vi "Standard Engine.vi"(8 "error in":errorcluster, 11 "Engine Process Init Data":T1) -> (0 "error out":errorcluster)   [LabVIEW 2013, in "Standard Engine Runtime.lvclass"]
uses:
  Standard Engine Runtime.lvclass
  Engine Process Init Data.ctl
  Commands.ctl
  Engine Config Data.ctl
  Configuration/Standard Engine Configuration.lvclass
  <vilib>/NI/Tag Bus Module Framework/runtime/TBM module execution interface.lvclass
  <vilib>/NI/Tag Bus Module Framework/module configuration/TBM module configuration.lvclass
  <vilib>/NI/Module Execution Interface/Engine Runtime/Execution States.ctl
  <vilib>/Platform/TimedLoop/XDataNode/timing_clust.ctl
  <vilib>/Platform/TimedLoop/XDataNode/nitl_modes.ctl
  <vilib>/Platform/TimedLoop/XDataNode/wakeup.ctl
  <vilib>/NI/Module Timing Source/timing source/TBM timing source.lvclass/TBM timing source.ctl
  <vilib>/NI/Module Timing Source/timing source/TBM timing source.lvclass
  <vilib>/NI/Tag Bus/table/transfer table data.vi
  Module Execution Decimation.vi
  Error Handler.vi
  <vilib>/Utility/error.llb/Clear Errors.vi
  Delete Module Index.vi
  <vilib>/platform/TimedLoop/XDataNode/XDataNode.xnode
  <vilib>/NI/Module Execution Interface/Engine Runtime/Engine Runtime Interface.lvclass
  <vilib>/Platform/TimedLoop/XDataNode/XDNodeRunTimeDep.lvlib
panel:
  out "late?":bool
  out "iterations":i32
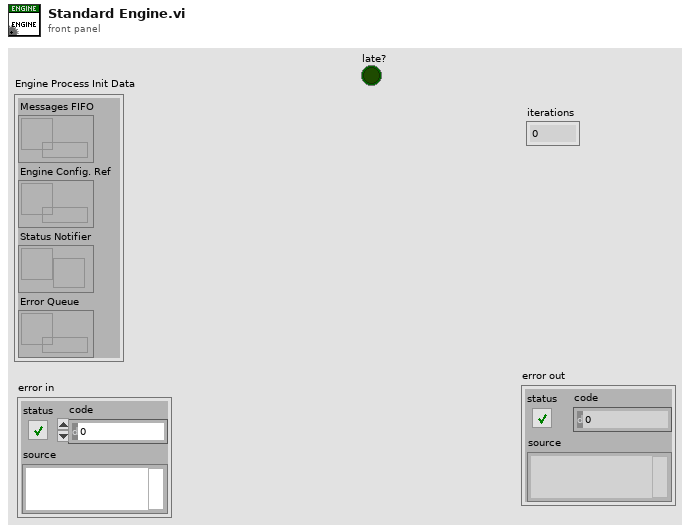
[diagram p1: front panel]
types:
  T1 = typedef "Standard Engine Runtime.lvclass/Engine Process Init Data.ctl" = cluster{"Messages FIFO":refnum<k33>, "Engine Config. Ref":refnum<data-value>, "Status Notifier":refnum<notifier>, "Error Queue":refnum<queue>}
  T2 = typedef "Engine Runtime Interface.lvclass/Execution States.ctl" = enum16{"Initializing", "Paused (Initialized)", "Running", "Set Safe Outputs", "Uninitializing", "Stopped (Uninitialized)", "Error (Uninitialized)", "Safe State (Uninitialized)", "Closed"}
  T3 = typedef "Standard Engine Runtime.lvclass/Commands.ctl" = enum16{"Initialize", "Start", "Pause", "Safe State", "Normal", "Stop", "Shutdown"}
  T4 = typedef "XDNodeRunTimeDep.lvlib/timing_clust.ctl" = cluster{"Expected End [f-1]":u64, "Actual End [f-1]":u64, "Finished Late? [f-1]":bool, "Expected End [i-1]":u64, "Actual End [i-1]":u64, "Finished Late? [i-1]":bool, "Expected Start [i]":u64, "Actual Start [i]":u64, "Expected Start [f]":u64, "Actual Start [f]":u64, "Source Name":string, "Structure Name":string, "Period":i64, "Deadline":i64, "Offset":i64, "Start":i64, "Priority":i32, "Timeout":i32, "Mode":T5, "Wakeup Reason":T6, "Error":errorcluster, "Source Type":string, "Secondary Source Type":string, "Global End Time":u64, "Global Start Time":u64, "Frame Duration":u64, "Iteration Duration":u64, "Assigned CPU":i32, "I/O Scan Engine Mode":u32}
  T5 = typedef "XDNodeRunTimeDep.lvlib/nitl_modes.ctl" = enum32{"No Change", "Process missed periods, maintain original phase", "Discard missed periods, maintain original phase", "Process missed periods, ignore original phase", "Discard missed periods, ignore original phase"}
  T6 = typedef "XDNodeRunTimeDep.lvlib/wakeup.ctl" = enum32{"Normal", "Aborted", "Asynchronous wakeup", "Timing source error", "Timed loop error", "Timeout"}
  T7 = typedef "Standard Engine Runtime.lvclass/Engine Data.ctl" = cluster{"Loop Info":T8, "Main Tag Data":T9, "Module Info":T10, "Safe State?":bool, "engine timing source":refnum<class "TBM timing source.lvclass">}
  T8 = typedef "Standard Engine Configuration.lvclass/Loop Info.ctl" = cluster{"Processor":i32, "Priority":i32}
  T9 = typedef "tag bus.lvlib/data table.lvlib/data table.ctl" = cluster{"Double":dbl[], "Single":sgl[], "I64":i64[], "I32":i32[], "I16":i16[], "I8":i8[], "U64":u64[], "U32":u32[], "U16":u16[], "U8":u8[], "Boolean":bool[], "String":string[], "Array of Double":cluster{"DBL Array":dbl[]}[], "Array of Single":cluster{"SGL Array":sgl[]}[], "Array of I64":cluster{"I64 Array":i64[]}[], "Array of I32":cluster{"I32 Array":i32[]}[], "Array of I16":cluster{"I16 Array":i16[]}[], "Array of I8":cluster{"I8 Array":i8[]}[], "Array of U64":cluster{"U64 Array":u64[]}[], "Array of U32":cluster{"U32 Array":u32[]}[], "Array of U16":cluster{"U16 Array":u16[]}[], "Array of U8":cluster{"U8 Array":u8[]}[], "Array of Boolean":cluster{"Boolean Array":bool[]}[], "Array of String":cluster{"String Array":string[]}[]}
  T10 = typedef "Standard Engine Runtime.lvclass/Module Execution Info.ctl" = cluster{"Tag Bus Modules":refnum<class "TBM module execution interface.lvclass">[], "Execute?":bool[], "Input Method Indices":i32[], "Process Method Indices":i32[], "Output Method Indices":i32[], "Input Transfer Specifications":T11[], "Parameter Transfer Specifications":T11[], "Result Transfer Specifications":T11[], "Output Transfer Specifications":T11[], "Module Errors":errorcluster[], "Module Decimation":T14[], "Module Decimation Indices":i32[], "Error Queue":refnum<queue>, "Module Error Configuration":T15[]}
  T11 = typedef "Standard Engine Runtime.lvclass/Data Table with Transfer Spec.ctl" = cluster{"Data Table":T9, "Transfer Specification":T12[]}
  T12 = typedef "tag bus.lvlib/data table.lvlib/transfer specification.ctl" = cluster{"data type":T13, "sink indices":i32[], "source indices":i32[]}
  T13 = typedef "tag bus.lvlib/tag descriptor.lvclass/Data Type.ctl" = enum16{"Double", "Single", "I64", "I32", "I16", "I8", "U64", "U32", "U16", "U8", "Boolean", "String", "Array of Double", "Array of Single", "Array of I64", "Array of I32", "Array of I16", "Array of I8", "Array of U64", "Array of U32", "Array of U16", "Array of U8", "Array of Boolean", "Array of String"}
  T14 = typedef "Standard Engine Configuration.lvclass/Module Decimation.ctl" = cluster{"Decimation":u16, "Offset":u16}
  T15 = typedef "Standard Engine Configuration.lvclass/Module Error Configuration.ctl" = cluster{"Module Error Configuration":T16[]}
  T16 = typedef "Standard Engine Configuration.lvclass/Error Actions By Category.ctl" = cluster{"error classification":T17, "Error Actions":T18[]}
  T17 = typedef "TBM module execution interface.lvclass/error classification.ctl" = enum16{"unknown", "none", "trivial", "recoverable", "critical"}
  T18 = typedef "Standard Engine Configuration.lvclass/Error Actions.ctl" = enum16{"Clear", "Notify", "Stop Component", "Stop Engine", "Safe State", "Attempt Recovery"}
  T19 = typedef "Standard Engine Runtime.lvclass/Engine Config Data.ctl" = cluster{"Engine Configuration":refnum<class "Standard Engine Configuration.lvclass">, "Modules":refnum<class "TBM module execution interface.lvclass">[], "Module Configurations":refnum<class "TBM module configuration.lvclass">[]}
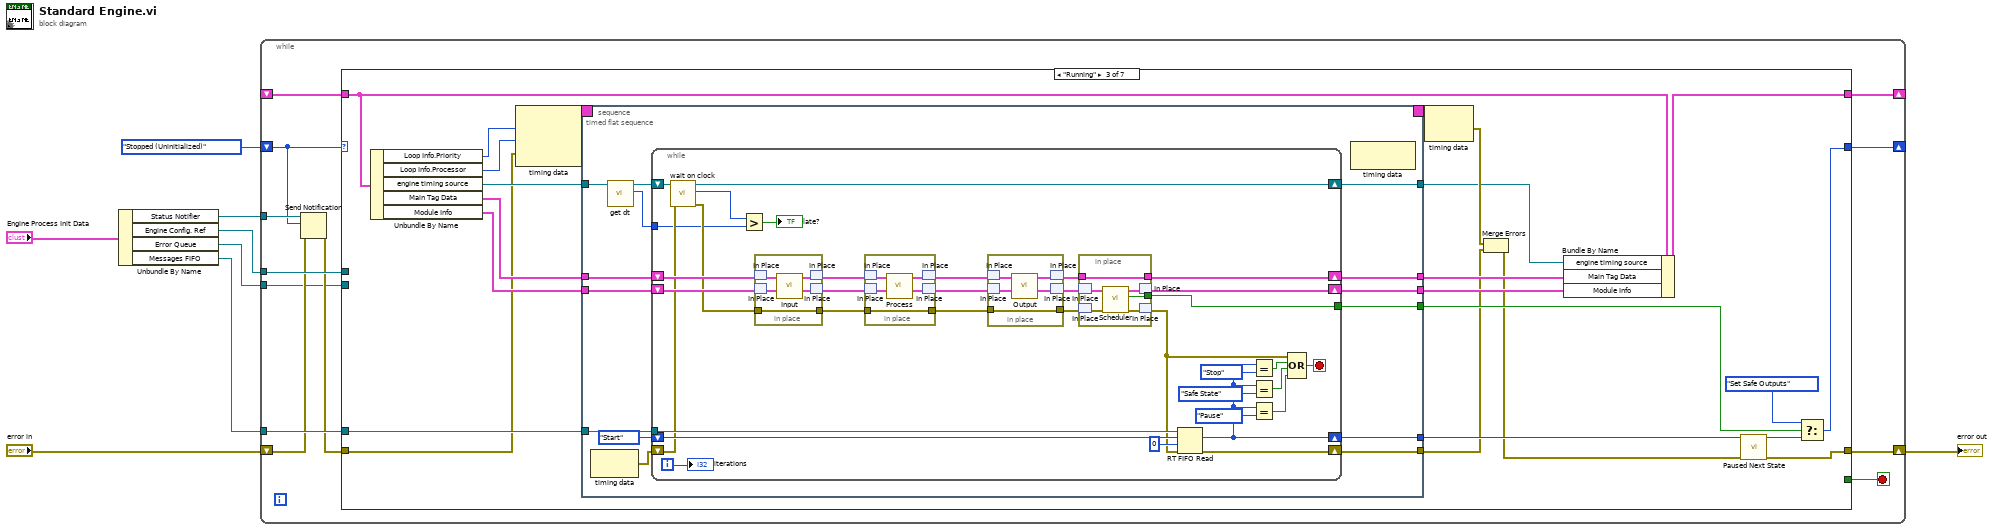
[diagram p0: block diagram]
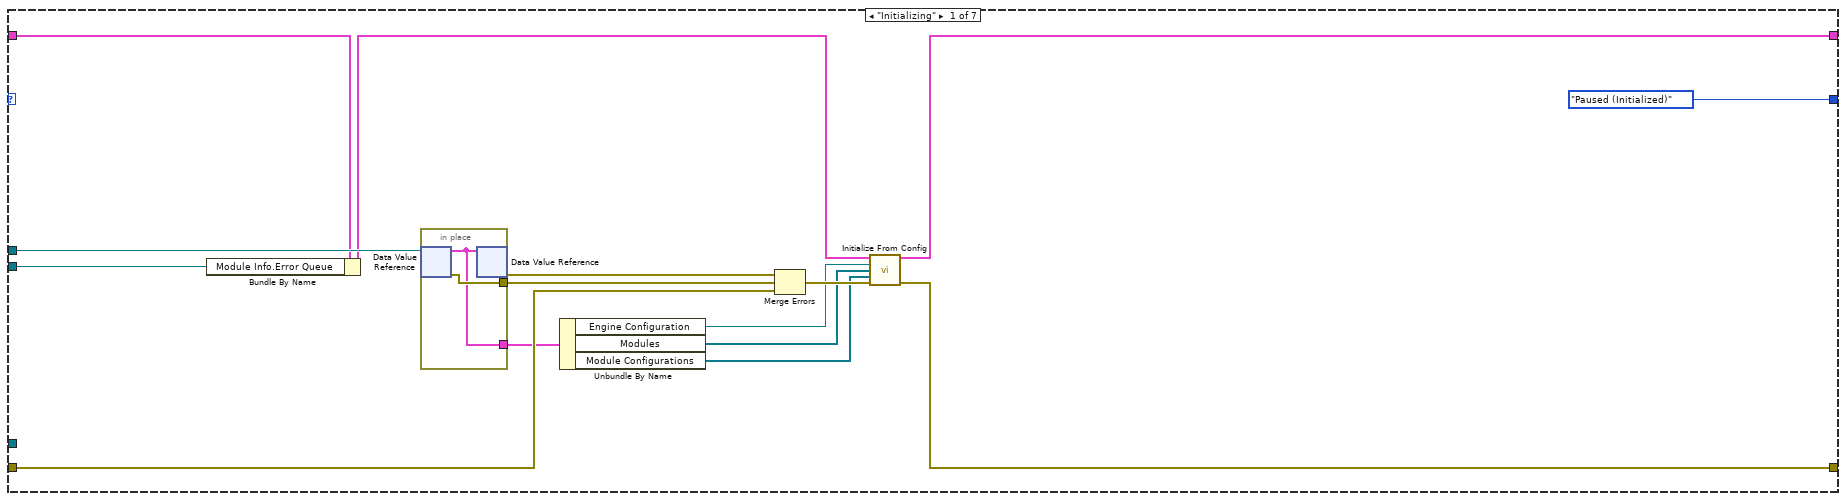
[diagram p2: hidden frame]
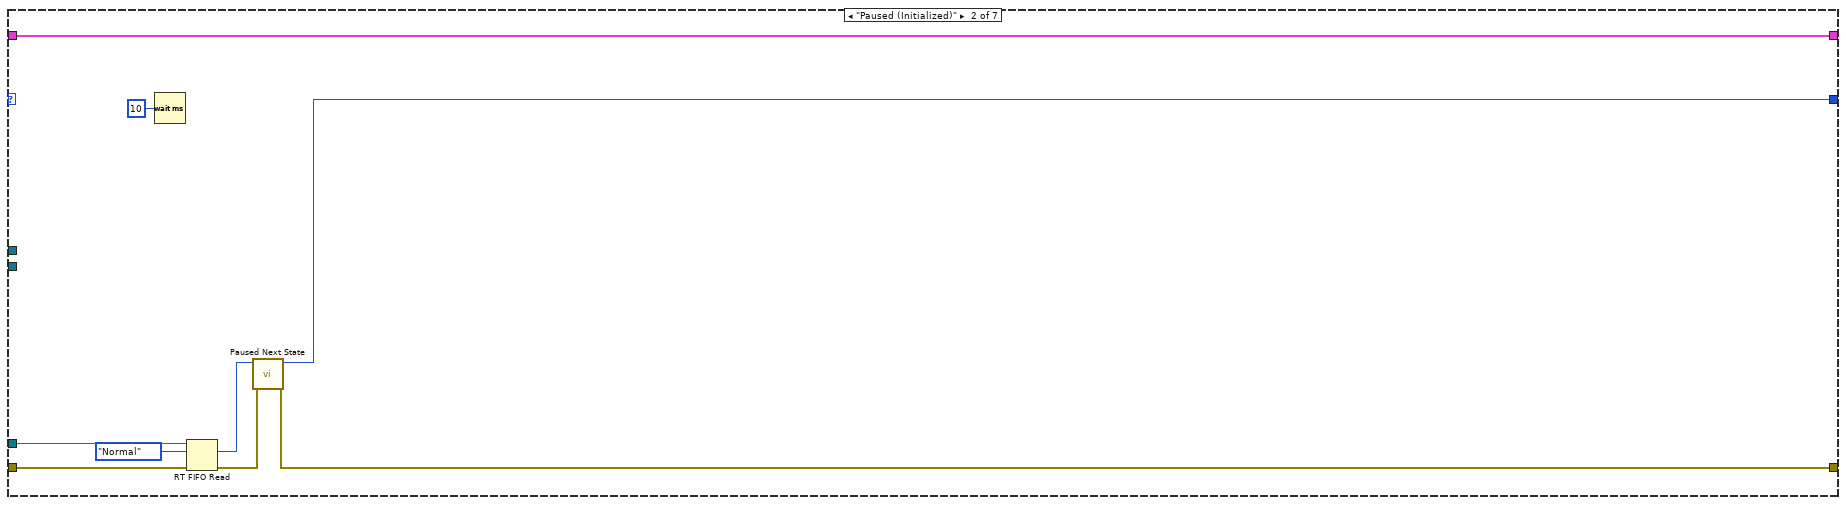
[diagram p3: hidden frame]
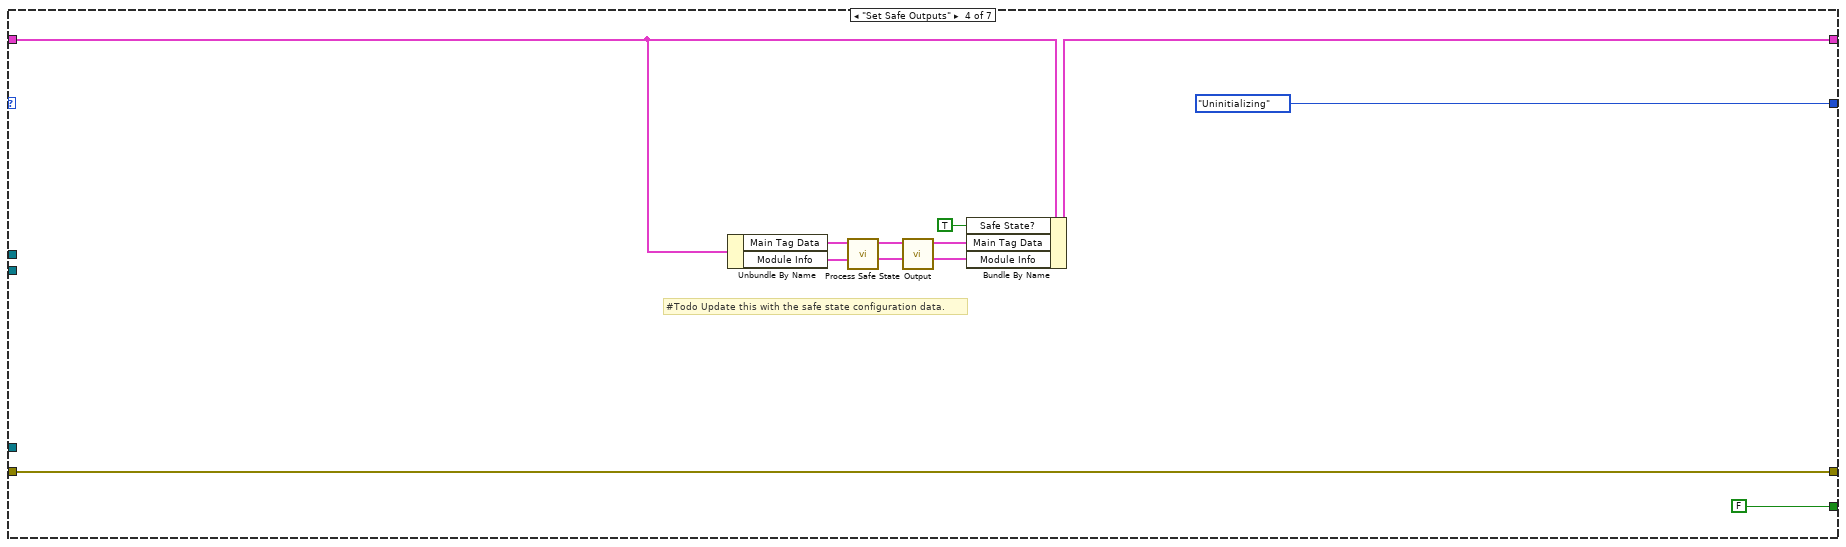
[diagram p4: hidden frame]
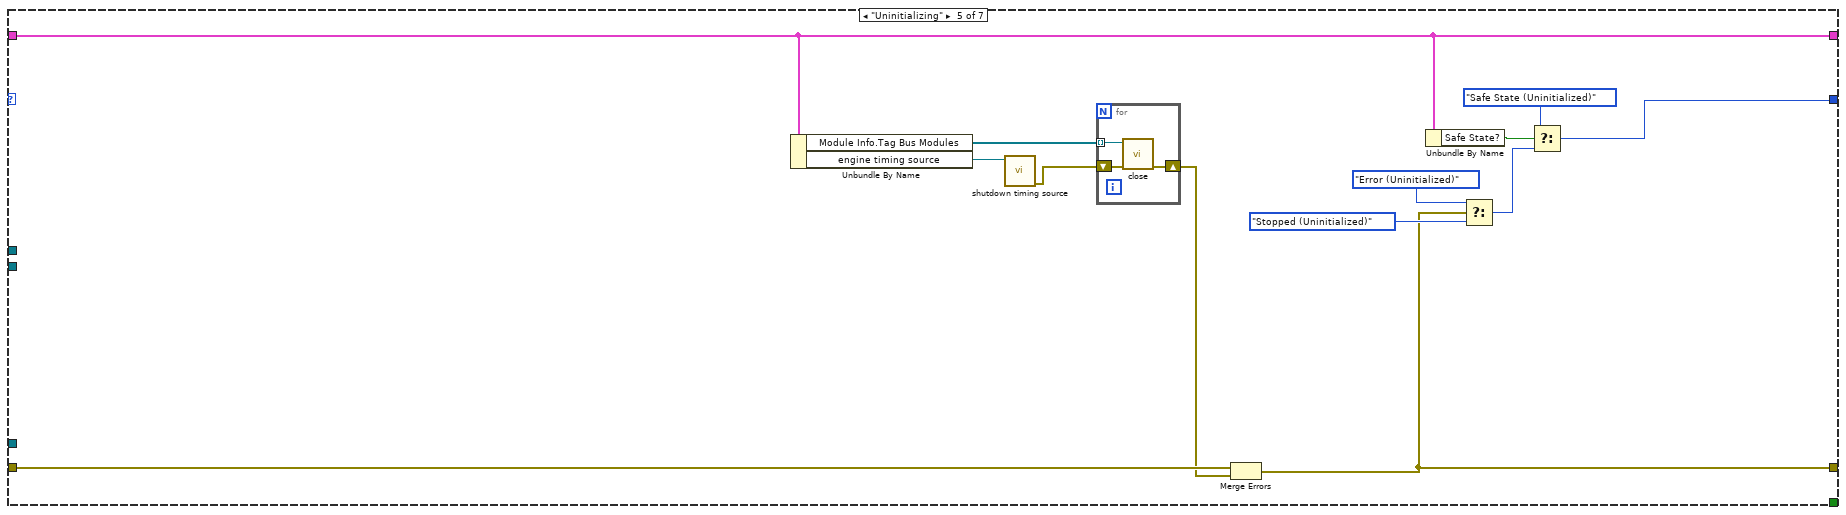
[diagram p5: hidden frame]
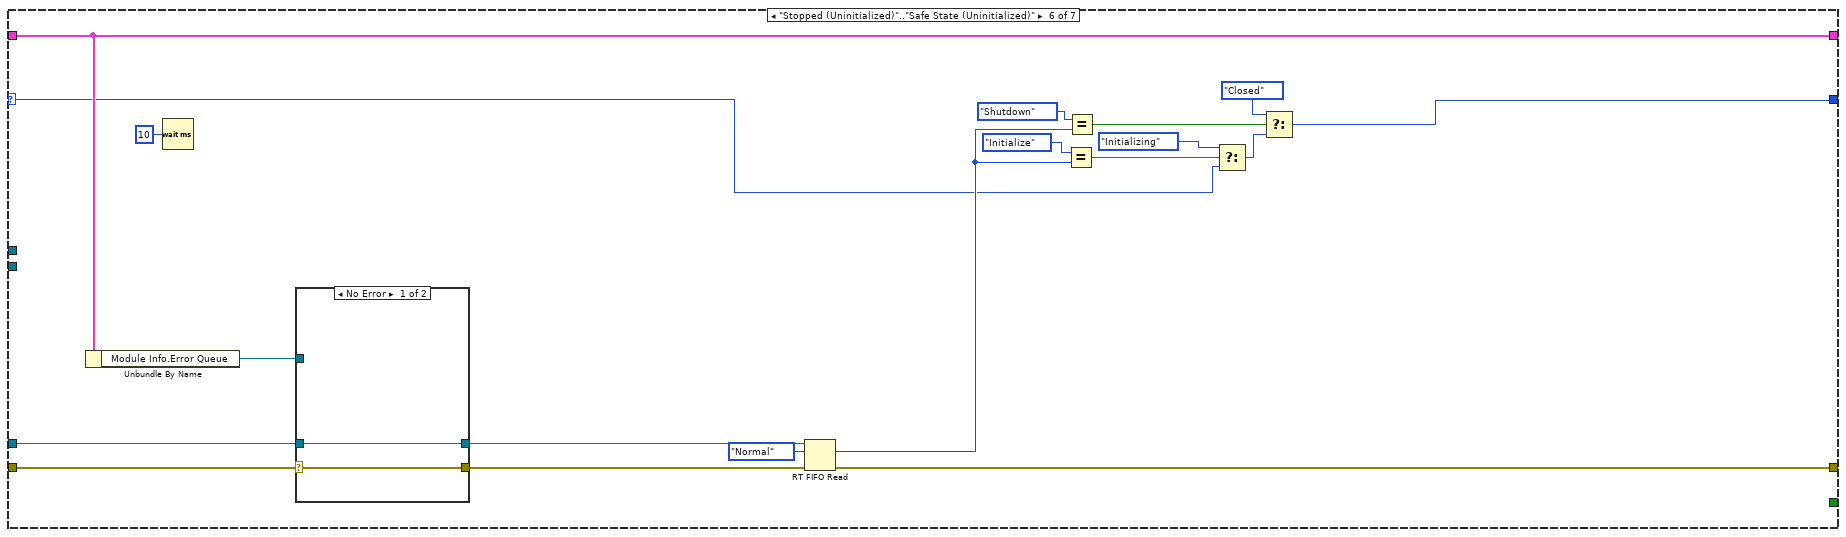
[diagram p6: hidden frame]
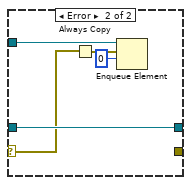
[diagram p7: hidden frame]
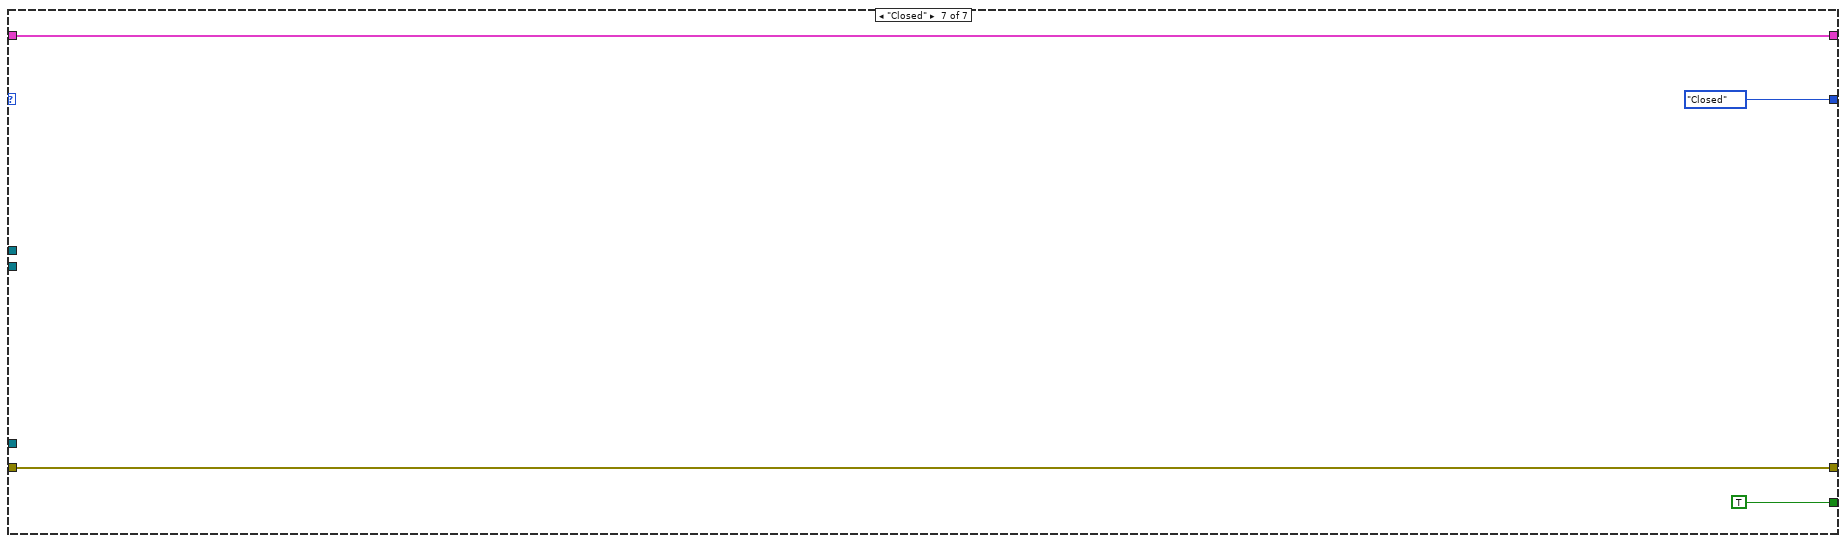
[diagram p8: hidden frame]
diagram:
  n1 = Unbundle By Name("Engine Process Init Data") -> ("Status Notifier"=w6:refnum<notifier>, "Engine Config. Ref"=w5:refnum<data-value>, "Error Queue"=w2:refnum<queue>, "Messages FIFO"=w4:refnum<k33>)
  n2 = while {
    shift-right: [w17] -> _
    shift-left: Execution_States."Stopped (Uninitialized)" ("States") -> [w12]
    shift-right: [w18] -> _
    shift-left: _ -> [w20]
    shift-right: [w19] -> w7
    shift-left: "error in" -> [w11]
    tunnel: w4 -> [w16]
    tunnel: w5 -> [w14]
    tunnel: w6 -> [w13]
    tunnel: w2 -> [w9]
    stop <- w15 stop-if-true
    n3 = Send Notification(notification=w12, notifier=w13, error in (no error)=w11) -> (error out=w10:errorcluster)  [unwired: 1 out]
    n4 = case shown="\"Running\"" w12 {
      selector: w12 -> [_ _ _ _ _ w189 _]
      tunnel: w20 -> [w24 w46 w55 w166 w183 w191 w215]
      tunnel: w10 -> [w32 w45 w51 w171 w174 w194 w217]
      tunnel: [w21 w39 w62 w171 w172 w201 w217] -> w19
      tunnel: [w30 w46 w64 w168 w183 w191 w215] -> w18
      tunnel: [Execution_States."Paused (Initialized)" ("States") w43 w58 Execution_States."Uninitializing" ("States") w177 w203 Execution_States."Closed" ("States")] -> w17
      tunnel: w16 -> [_ w38 w69 _ _ w193 _]
      tunnel: [_ _ _ FALSE _ _ TRUE] -> w15
      tunnel: w14 -> [w27 _ _ _ _ _ _]
      tunnel: w9 -> [w23 _ _ _ _ _ _]
      frame "Initializing" {
        n5 = Bundle By Name(cluster=w24, "Module Info.Error Queue"=w23) -> (w22:T7)
        n6 = in-place {
          in-place-border: [w37] -> w33
          in-place-border: [w36] -> w31
          n7 = in-place-dvr #1(w27) -> (w36:T19, w37:errorcluster)
          n8 = in-place-dvr #1(w36) -> (w34:errorcluster)  [unwired: 1 out]
        }
        n9 = Unbundle By Name(w31) -> ("Engine Configuration"=w28:refnum<class "Standard Engine Configuration.lvclass">, "Modules"=w26:refnum<class "TBM module execution interface.lvclass">[], "Module Configurations"=w25:refnum<class "TBM module configuration.lvclass">[])
        n10 = Merge Errors(w34, w33, w32) -> (w29:errorcluster)
        n11 = call "Initialize From Config.vi"("Engine Data"=w22, "Engine Configuration"=w28, "Modules"=w26, "Module Configurations"=w25, "error in"=w29) -> ("Engine Data Out"=w30:T7, "error out"=w21:errorcluster)  [unwired: 9 in]
      }
      frame "Paused (Initialized)" {
        n12 = Wait (ms)(milliseconds to wait=u32 10) -> ()  [unwired: 1 out]
        n13 = RT FIFO Read(0:w38, 1:Commands."Normal" ("Commands"), 3:w45) -> (9:w42:T3, 11:w41:errorcluster)  [unwired: 1 in, 3 out]
        n14 = call "Paused Next State.vi"("error in"=w41, "Command"=w42) -> ("error out"=w39:errorcluster, "State"=w43:T2)  [unwired: 8 in]
      }
      frame "Running" {
        n15 = Unbundle By Name(w55) -> ("Loop Info.Priority"=w49:i32, "Loop Info.Processor"=w53:i32, "engine timing source"=w52:refnum<class "TBM timing source.lvclass">, "Main Tag Data"=w68:T9, "Module Info"=w67:T10)
        n16 = node-c288(w49, w53, w51) -> (w48:T4)
        n17 = timed-sequence {
          timing: w48 -> [_]
          timing-out: [_] -> w47
          tunnel: w69 -> [w79]
          tunnel: w68 -> [w78]
          tunnel: w67 -> [w77]
          tunnel: [w76] -> w66
          tunnel: [w75] -> w65
          tunnel: [w74] -> w63
          tunnel: [w73] -> w60
          tunnel: [w72] -> w57
          tunnel: w52 -> [w71]
          tunnel: [w70] -> w50
          n18 = timed-flat-sequence {
            tunnel: w79 -> [w93]
            tunnel: w78 -> [w91]
            tunnel: w77 -> [w90]
            tunnel: [w89] -> w76
            tunnel: [w88] -> w75
            tunnel: [w87] -> w74
            tunnel: [w86] -> w73
            tunnel: [w83] -> w72
            tunnel: w71 -> [w85]
            tunnel: [w82] -> w70
            n19 = node-c288() -> (w84:errorcluster)  [unwired: 1 in]
            n20 = call <vilib>:"get dt.vi"("timing source in"=w85) -> ("dt"=w80:u32, "timing source out"=w81:refnum<class "TBM timing source.lvclass">)  [unwired: 9 in]
            n21 = while {
              tunnel: w93 -> [w114]
              shift-right: [w122] -> w87
              shift-left: Commands."Start" ("Commands") -> [w131]
              shift-right: [w111] -> w89
              shift-left: w91 -> [w129]
              shift-right: [w123] -> w88
              shift-left: w90 -> [w128]
              tunnel: [w109] -> w86
              shift-right: [w113] -> w83
              shift-left: w84 -> [w102]
              shift-right: [w100] -> w82
              shift-left: w81 -> [w103]
              tunnel: w80 -> [w98]
              i -> [w108]
              stop <- w115 stop-if-true
              n22 = call-dynamic "wait on clock.vi"("error in"=w102, "timing source in"=w103) -> ("error out"=w101:errorcluster, "ticks since last call"=w99:u32, "timing source out"=w100:refnum<class "TBM timing source.lvclass">)  [unwired: 7 in]
              n23 = Greater?(x=w99, y=w98) -> (0:→"late?":bool)
              n24 = in-place {
                in-place-border: w101 -> [w148]
                in-place-border: [w148] -> w106
                n25 = in-place-match #2(w129) -> (w152:T9)
                n26 = in-place-match #3(w128) -> (w151:T10)
                n27 = call "Input.vi"("Module Info In"=w151, "Engine Tags In"=w152) -> ("Module Info Out"=w149:T10, "Engine Tags Out"=w150:T9)  [unwired: 8 in]
                n28 = in-place-match #2(w150) -> (w127:T9)
                n29 = in-place-match #3(w149) -> (w126:T10)
              }
              n30 = in-place {
                in-place-border: w106 -> [w143]
                in-place-border: [w143] -> w105
                n31 = in-place-match #4(w127) -> (w146:T9)
                n32 = in-place-match #5(w126) -> (w147:T10)
                n33 = call "Process.vi"("Module Info In"=w147, "Engine Tags In"=w146) -> ("Module Info Out"=w144:T10, "Engine Tags Out"=w145:T9)  [unwired: 8 in]
                n34 = in-place-match #4(w145) -> (w107:T9)
                n35 = in-place-match #5(w144) -> (w125:T10)
              }
              n36 = in-place {
                in-place-border: w105 -> [w138]
                in-place-border: [w138] -> w104
                n37 = in-place-match #6(w107) -> (w142:T9)
                n38 = in-place-match #7(w125) -> (w140:T10)
                n39 = call "Output.vi"("Module Info In"=w140, "Engine Tags In"=w142) -> ("Module Info Out"=w139:T10, "Engine Tags Out"=w141:T9)  [unwired: 8 in]
                n40 = in-place-match #6(w141) -> (w110:T9)
                n41 = in-place-match #7(w139) -> (w124:T10)
              }
              n42 = in-place {
                in-place-border: [w135] -> w111
                in-place-border: w110 -> [w135]
                in-place-border: [w132] -> w109
                n43 = in-place-match #8(w124) -> (w134:T10)
                n44 = in-place-match #9(w104) -> (w137:errorcluster)
                n45 = call "Scheduler.vi"("error in"=w137, "Module Info In"=w134) -> ("error out"=w136:errorcluster, "Safe State?"=w132:bool, "Module Info Out"=w133:T10)  [unwired: 7 in]
                n46 = in-place-match #8(w133) -> (w123:T10)
                n47 = in-place-match #9(w136) -> (w112:errorcluster)
              }
              n48 = RT FIFO Read(0:w114, 1:w131, 2:0 ("timeout in ms (0)"), 3:w112) -> (9:w122:T3, 11:w113:errorcluster)  [unwired: 3 out]
              n49 = Equal?(x=w122, y=Commands."Stop") -> (x = y?=w118:bool)
              n50 = Equal?(x=w122, y=Commands."Safe State") -> (x = y?=w117:bool)
              n51 = Equal?(x=w122, y=Commands."Pause") -> (x = y?=w116:bool)
              n52 = Compound Arithmetic op=OR(w112, w118, w117, w116) -> (w115:bool)
              "iterations" <- w108
            }
            n53 = node-c288() -> ()  [unwired: 1 in, 1 out]
          }
        }
        n54 = node-c288(w47) -> (w54:errorcluster)
        n55 = Merge Errors(w54, w57) -> (w56:errorcluster)
        n56 = Bundle By Name(cluster=w55, "engine timing source"=w50, "Main Tag Data"=w66, "Module Info"=w65) -> (w64:T7)
        n57 = call "Paused Next State.vi"("error in"=w56, "Command"=w63) -> ("error out"=w62:errorcluster, "State"=w61:T2)  [unwired: 8 in]
        n58 = Select(t=Execution_States."Set Safe Outputs", s=w60, f=w61) -> (s? t:f=w58:T2)
      }
      frame "Set Safe Outputs" {
        # "#Todo Update this with the safe state configuration data."
        n59 = Unbundle By Name(w166) -> ("Main Tag Data"=w165:T9, "Module Info"=w164:T10)
        n60 = call "Process Safe State.vi"("Module Info In"=w164, "Engine Tags In"=w165) -> ("Module Info Out"=w162:T10, "Engine Tags Out"=w163:T9)  [unwired: 8 in]
        n61 = call "Output.vi"("Module Info In"=w162, "Engine Tags In"=w163) -> ("Module Info Out"=w160:T10, "Engine Tags Out"=w161:T9)  [unwired: 8 in]
        n62 = Bundle By Name(cluster=w166, "Safe State?"=TRUE, "Main Tag Data"=w161, "Module Info"=w160) -> (w168:T7)
      }
      frame "Uninitializing" {
        n63 = Unbundle By Name(w183) -> ("Module Info.Tag Bus Modules"=w184:refnum<class "TBM module execution interface.lvclass">[], "engine timing source"=w176:refnum<class "TBM timing source.lvclass">)
        n64 = call-dynamic "shutdown timing source.vi"("timing source in"=w176) -> ("error out"=w175:errorcluster)  [unwired: 9 in, 1 out]
        n65 = for {
          tunnel: w184 -> [w187] mode=indexing
          shift-right: [w185] -> w173
          shift-left: w175 -> [w186]
          n66 = call-dynamic "close.vi"("error in"=w186, "module in"=w187) -> ("error out"=w185:errorcluster)  [unwired: 9 in]
        }
        n67 = Merge Errors(w174, w173) -> (w172:errorcluster)
        n68 = Unbundle By Name(w183) -> ("Safe State?"=w182:bool)
        n69 = Select(t=Execution_States."Error (Uninitialized)" ("States"), s=w172, f=Execution_States."Stopped (Uninitialized)" ("States")) -> (s? t:f=w178:T2)
        n70 = Select(t=Execution_States."Safe State (Uninitialized)" ("States"), s=w182, f=w178) -> (s? t:f=w177:T2)
      }
      frame "Stopped (Uninitialized)".."Safe State (Uninitialized)" {
        n71 = Unbundle By Name(w191) -> ("Module Info.Error Queue"=w190:refnum<queue>)
        n72 = Wait (ms)(milliseconds to wait=u32 10) -> ()  [unwired: 1 out]
        n73 = case shown="No Error" w194 {
          selector: w194 -> [w207 w211]
          tunnel: w193 -> [w208 w213]
          tunnel: [w208 w213] -> w192
          tunnel: [w207 _] -> w188
          tunnel: w190 -> [_ w212]
          frame No Error {
          }
          frame Error {
            n74 = Always Copy(1:w211) -> (0:w210:errorcluster)
            n75 = Enqueue Element(queue=w212, element=w210, timeout in ms (-1)=0) -> ()  [unwired: 1 in, 3 out]
          }
        }
        n76 = RT FIFO Read(0:w192, 1:Commands."Normal" ("Commands"), 3:w188) -> (9:w206:T3, 11:w201:errorcluster)  [unwired: 1 in, 3 out]
        n77 = Equal?(x=Commands."Initialize" ("Commands"), y=w206) -> (x = y?=w205:bool)
        n78 = Equal?(x=Commands."Shutdown" ("Commands"), y=w206) -> (x = y?=w200:bool)
        n79 = Select(t=Execution_States."Initializing" ("States"), s=w205, f=w189) -> (s? t:f=w204:T2)
        n80 = Select(t=Execution_States."Closed" ("States"), s=w200, f=w204) -> (s? t:f=w203:T2)
      }
      frame "Closed" {
      }
    }
  }
  "error out" <- w7
